vi "Lab03.vi"() -> ()   [LabVIEW 2022 SP3]
uses:
  <vilib>/numeric/Random Number (Range) DBL.vi
panel:
  out "second subarray":dbl[](array[numeric])
  out "first subarray":dbl[](array[numeric])
  out "Ran2":dbl[](array[numeric])
  out "Ran1":dbl[](array[numeric])
  out "Waveform Graph":dbl[][](graph)
  in  "# of Periods":dbl
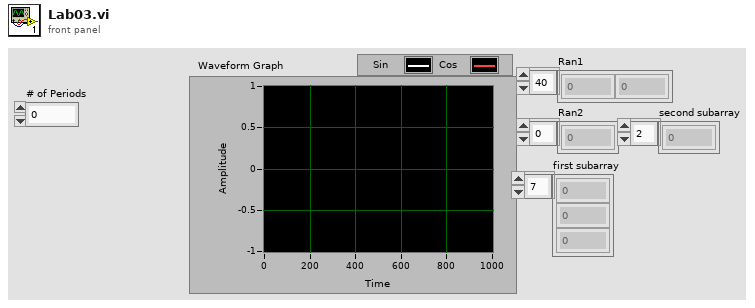
[diagram p1: front panel]
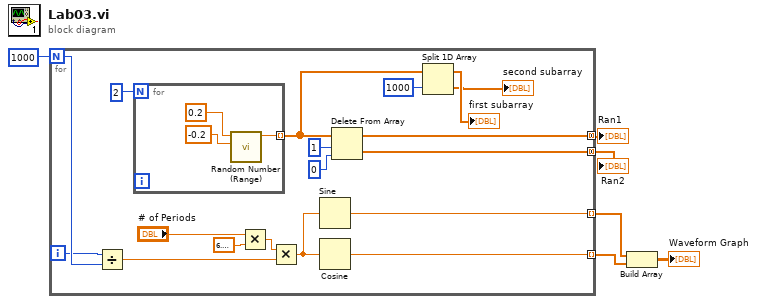
[diagram p0: block diagram]
diagram:
  n1 = for {
    N: 1000 -> [w22]
    tunnel: [w14] -> w2 mode=concatenating
    tunnel: [w13] -> w1 mode=concatenating
    tunnel: [w12] -> w4 mode=indexing
    tunnel: [w11] -> w5 mode=indexing
    i -> [w21]
    n2 = Divide(x=w21, y=w22) -> (x/y=w20:dbl)
    n3 = for {
      N: 2 -> [_]
      tunnel: [w25] -> w9 mode=indexing
      n4 = call-poly <vilib>:"Random Number (Range).vi"("lower bound (0)"=-0.2, "upper bound (100)"=0.2) -> ("number"=w25:dbl)  [unwired: 9 in]
    }
    n5 = Multiply(x="# of Periods", y=6.283185307179586) -> (x*y=w19:dbl)
    n6 = Multiply(x=w19, y=w20) -> (x*y=w18:dbl)
    n7 = Sine(x=w18) -> (sin(x)=w12:dbl)
    n8 = Cosine(x=w18) -> (cos(x)=w11:dbl)
    n9 = Delete From Array(array=w9, length=1, index=0) -> (deleted portion=w13:dbl[], array with subset deleted=w14:dbl[])
    n10 = Split 1D Array(array=w9, index=1000) -> (first subarray=→"first subarray":dbl[], second subarray=→"second subarray":dbl[])
  }
  "Ran1" <- w2
  "Ran2" <- w1
  n11 = Build Array(w4, w5) -> (→"Waveform Graph":dbl[][])
